vi "BuildHelpPath.vi"(1 "Help File Name":string="lvhelp.chm" caption="帮助文件名") -> (0 "Help File Path":path caption="帮助文件路径")   [LabVIEW 2018]
doc: "该VI将传入的文件名拼接至帮助目录，并返回完整路径。当未指定输入时，默认输入为LabVIEW的主帮助文件。"
panel:
  # "该VI将传入的文件名拼接至帮助目录，并返回\n完整路径。当未指定输入时，默认输入为LabVIEW的主帮助文件。"
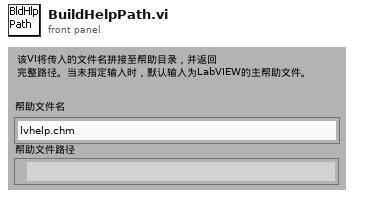
[diagram p1: front panel]
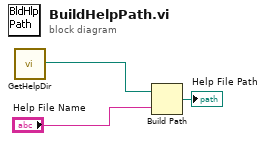
[diagram p0: block diagram]
diagram:
  n1 = call "GetHelpDir.vi"() -> ("help path"=w3:path)
  n2 = Build Path(base path=w3, name or relative path="Help File Name") -> (appended path=→"Help File Path":path)
